vi "score generator.vi"(2 "maximum":dbl=80.0, 4 "minimum":dbl=20.0) -> (0 "Array":i32[](array[numeric]))   [LabVIEW 2014]
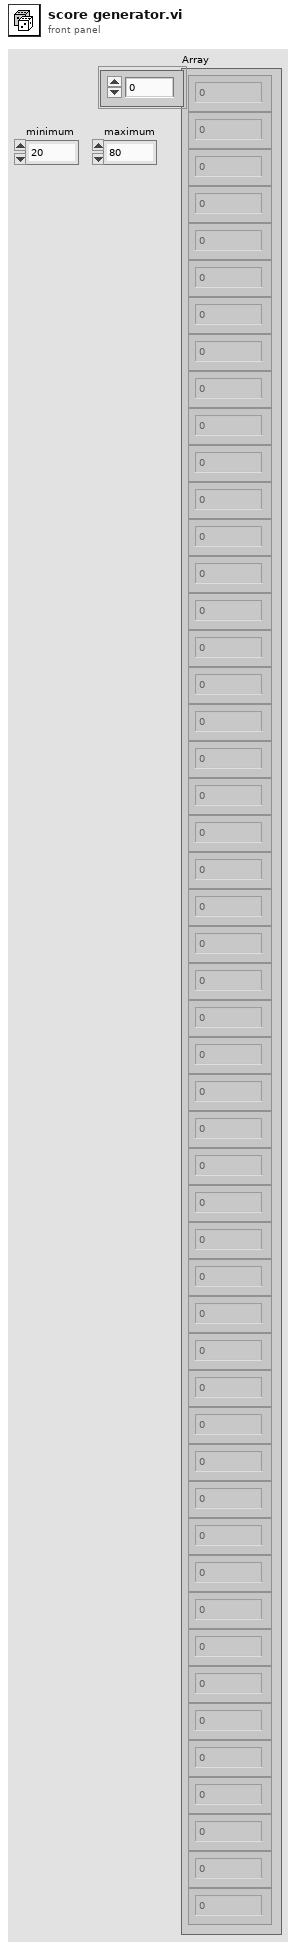
[diagram p1: front panel]
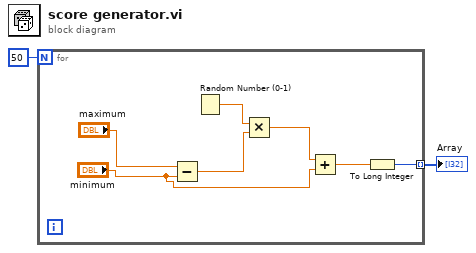
[diagram p0: block diagram]
diagram:
  n1 = for {
    N: 50 -> [_]
    tunnel: [w3] -> w1 mode=indexing
    n2 = Subtract(x="maximum", y="minimum") -> (x-y=w7:dbl)
    n3 = Random Number (0-1)() -> (number: 0 to 1=w8:dbl)
    n4 = Multiply(x=w8, y=w7) -> (x*y=w6:dbl)
    n5 = Add(x=w6, y="minimum") -> (x+y=w4:dbl)
    n6 = To Long Integer(number=w4) -> (32bit integer=w3:i32)
  }
  "Array" <- w1
